vi "drop_dbconn.vi"() -> (0 "错误输出":errorcluster, 8 "错误输入":errorcluster caption="错误输出")   [LabVIEW 2015]
uses:
  global/tcp_conn.vi
panel:
  # "调用本模块，自动销毁远程数据库连接"
  # "注：程序关闭时，请调用本模块销毁远程数据库连接"
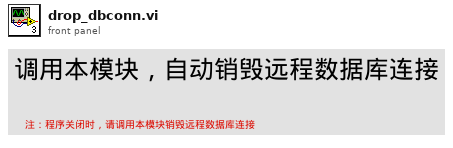
[diagram p1: front panel]
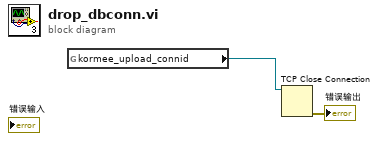
[diagram p0: block diagram]
diagram:
  n1 = global read "tcp_conn.vi" "kormee_upload_connid"() -> (w2:refnum<k5>)
  n2 = TCP Close Connection(connection ID=w2) -> (error out=→"错误输出":errorcluster)  [unwired: 2 in, 1 out]
